vi "Write Radio.vi"(8 "error in (no error)":errorcluster, 10 "Radio":dbl, 11 "Circulo in":refnum<class "Circulo.lvclass">) -> (0 "error out":errorcluster, 3 "Circulo out":refnum<class "Circulo.lvclass">)   [LabVIEW 2024, in "Circulo.lvclass"]
uses:
  Circulo.lvclass
  Circulo.lvclass/Circulo.ctl
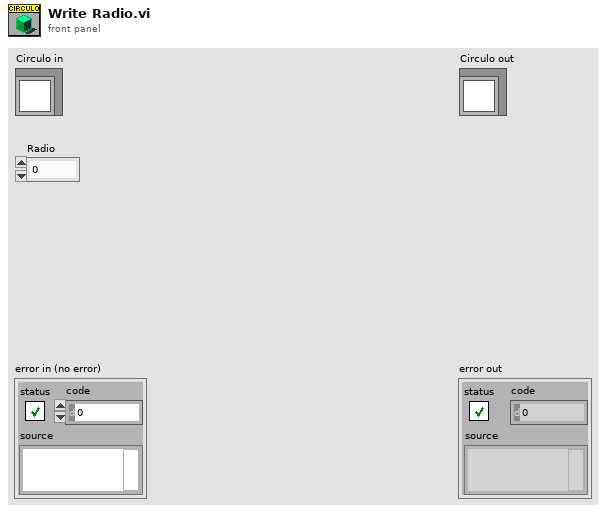
[diagram p1: front panel]
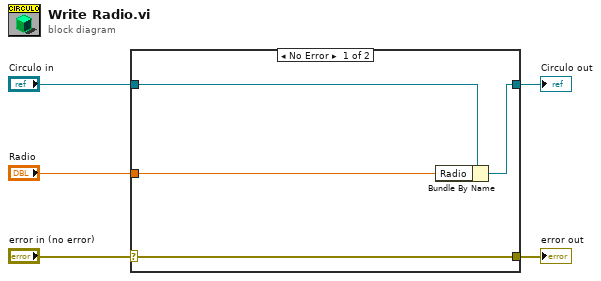
[diagram p0: block diagram]
diagram:
  n1 = case shown="No Error" "error in (no error)" {
    selector: "error in (no error)" -> [w9 w10]
    tunnel: [w9 w10] -> w4
    tunnel: [w7 w11] -> w2
    tunnel: "Circulo in" -> [w8 w11]
    tunnel: "Radio" -> [w6 _]
    frame No Error {
      n2 = Bundle By Name(cluster=w8, "Radio"=w6) -> (w7:refnum<class "Circulo.lvclass">)
    }
    frame Error {
    }
  }
  "error out" <- w4
  "Circulo out" <- w2
